vi "Fast_FID_Valve_Control.vi"(7 "Requested Position":T1=1 items=["", "Zero Air", "Calib 1", "Calib 2", "Measure"]) -> (0 "Error Message":string, 3 "Achieved Posn.":T1=1 items=["", "Zero Air", "Calib 1", "Calib 2", "Measure"])   [LabVIEW 2013]
uses:
  Sub VIs/ADAM Controls/Valco_valve_ph.ctl
  Anemometry/Anemometry Sub Vis/Controls/Post_Process.ctl
  Anemometry/Anemometry Sub Vis/Globals/Preference_global.vi
  Anemometry/Anemometry Sub Vis/Globals/Meas_global.vi
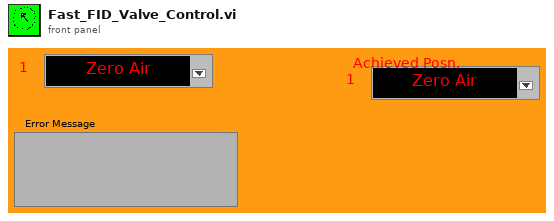
[diagram p1: front panel]
types:
  T1 = typedef "Valco_valve_ph.ctl" = u16
  T2 = typedef "Post_Process.ctl" = enum16{"Take New Data", "Post Process Raw Data File"}
  T3 = typedef "Server_Comms.ctl" = enum16{"Server Link Healthy", "Do Not Link To Server"}
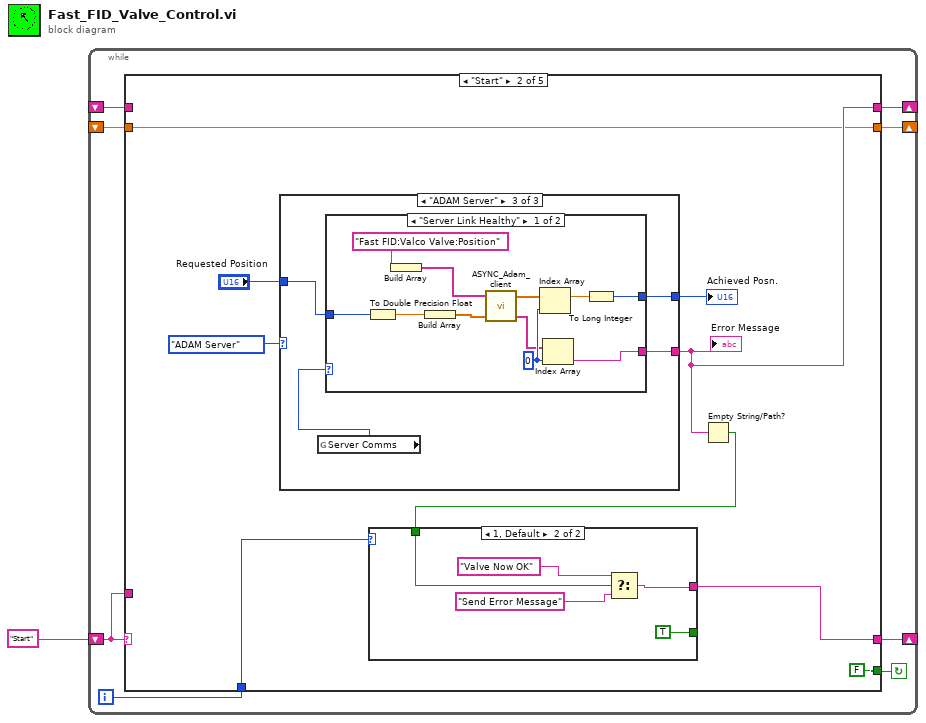
[diagram p0: block diagram]
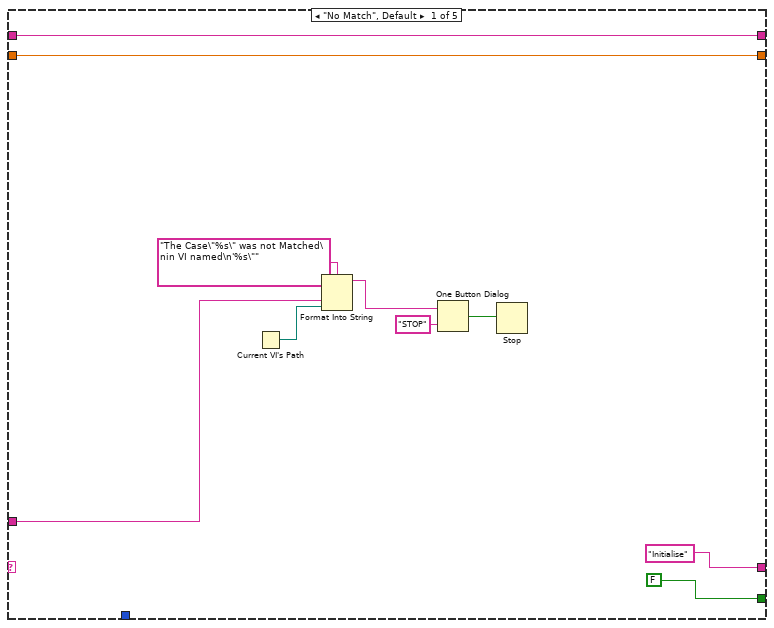
[diagram p2: hidden frame]
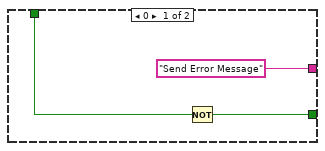
[diagram p3: hidden frame]
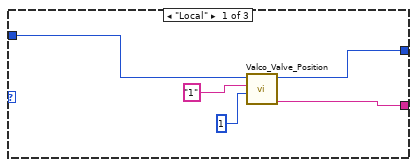
[diagram p4: hidden frame]
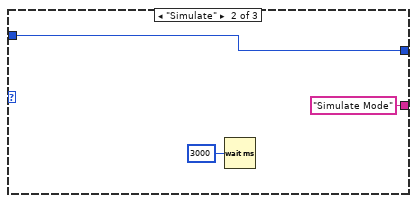
[diagram p5: hidden frame]
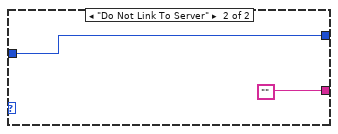
[diagram p6: hidden frame]
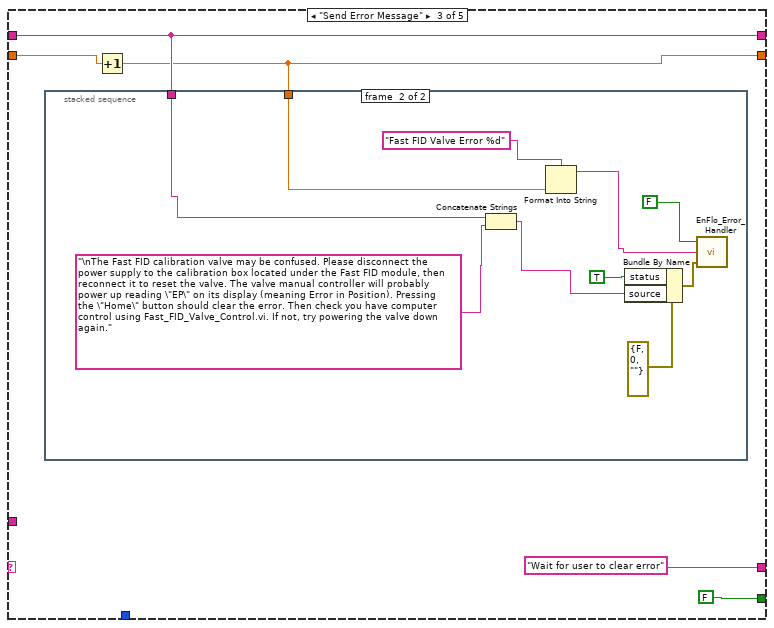
[diagram p7: hidden frame]
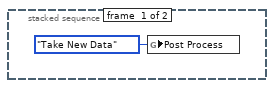
[diagram p8: hidden frame]
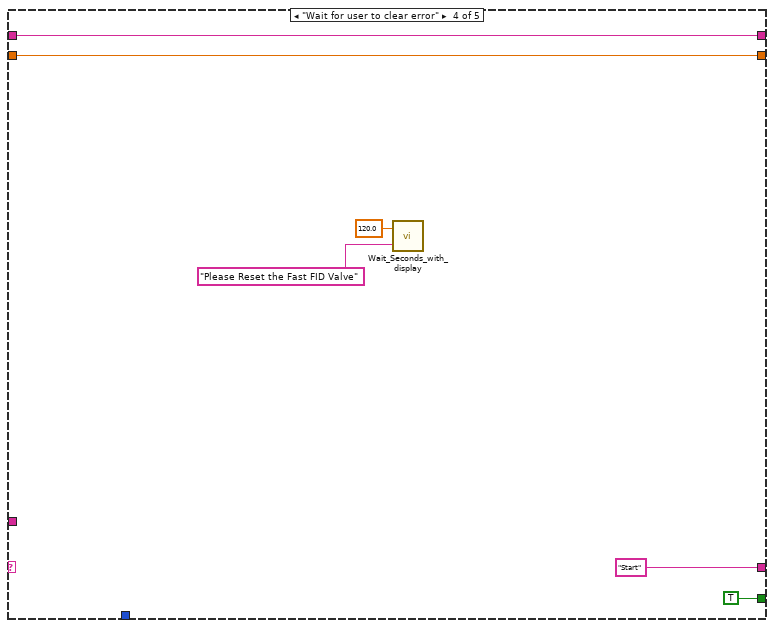
[diagram p9: hidden frame]
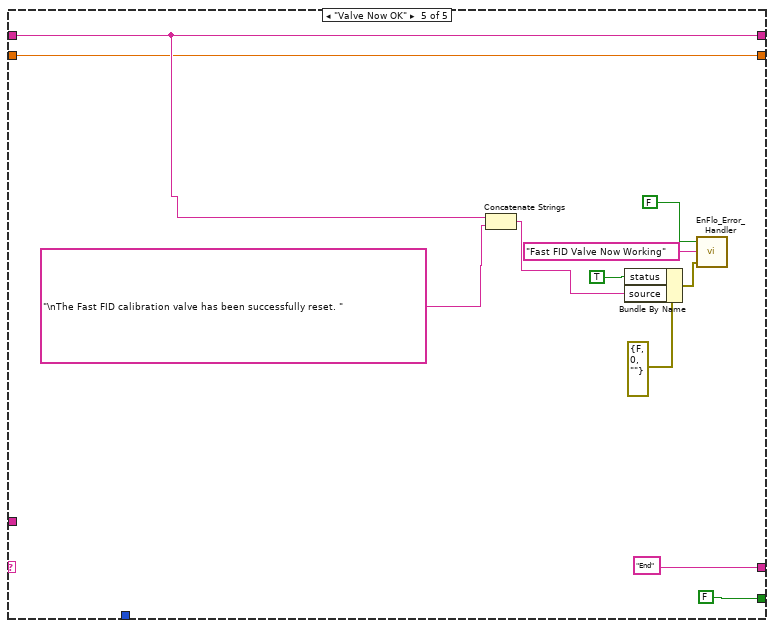
[diagram p10: hidden frame]
diagram:
  n1 = while {
    shift-left: "Start" -> [w7]
    shift-right: [w8] -> _
    shift-right: [w6] -> _
    shift-left: _ -> [w5]
    shift-right: [w2] -> _
    shift-left: _ -> [w3]
    i -> [w4]
    stop <- w9 continue-if-true
    n2 = case shown="\"Start\"" w7 {
      tunnel: [FALSE FALSE FALSE TRUE FALSE] -> w9
      tunnel: ["Initialise" w23 "Wait for user to clear error" "Start" "End"] -> w8
      tunnel: w7 -> [w14 _ _ _ _]
      tunnel: [w11 w26 w64 w80 w85] -> w6
      tunnel: w5 -> [w11 _ w64 w80 w85]
      tunnel: w4 -> [_ w25 _ _ _]
      tunnel: w3 -> [w10 w22 w63 w78 w84]
      tunnel: [w10 w22 w62 w78 w84] -> w2
      frame "No Match", Default {
        n3 = Current VI's Path() -> (path=w13:path)
        n4 = Format Into String(format string="The Case\"%s\" was not Matched\nin VI named\n'%s\"" ("Format String"), w14, w13) -> (resulting string=w17:string)  [unwired: 2 in, 1 out]
        n5 = One Button Dialog(message=w17, button name ("OK")="STOP") -> (true=w15:bool)
        n6 = Stop(stop? (T)=w15) -> ()
      }
      frame "Start" {
        n7 = case shown="\"ADAM Server\"" enum16{"Local", "ADAM Server", "Simulate"}."ADAM Server" ("Case Constant\n(See Context Help)") {
          tunnel: "Requested Position" -> [w40 w44 w48]
          tunnel: [w39 w44 w47] -> w28
          tunnel: [w38 "Simulate Mode" w46] -> w26
          frame "Local" {
            n8 = call "Valco_Valve_Position.vi"("Valve Number"=1, "Port Name"="1", "Requested Posn."=w40) -> ("Error Message"=w38:string, "Achieved Posn."=w39:T1)  [unwired: 1 in, 2 out]
          }
          frame "Simulate" {
            n9 = Wait (ms)(milliseconds to wait=u32 3000) -> ()  [unwired: 1 out]
          }
          frame "ADAM Server" {
            n10 = global read "Preference_global.vi" "Server Comms"() -> (w45:T3)
            n11 = case shown="\"Server Link Healthy\"" w45 {
              tunnel: w48 -> [w51 w61]
              tunnel: [w50 w61] -> w47
              tunnel: [w49 ""] -> w46
              frame "Server Link Healthy" {
                w59 = 0 ("Index")
                n12 = To Double Precision Float(number=w51) -> (double precision float=w54:dbl)
                n13 = Build Array("Fast FID:Valco Valve:Position") -> (w55:string[])
                n14 = Build Array(w54) -> (w56:dbl[])
                n15 = call "ASYNC_Adam_client.vi"("Values"=w56, "Channel Names"=w55) -> ("Scan Comments"=w58:string[], "Calibrated Units"=w57:dbl[])  [unwired: 1 in]
                n16 = Index Array(array=w57, index=w59) -> (element=w53:dbl)
                n17 = Index Array(array=w58, index=w59) -> (element=w49:string)
                n18 = To Long Integer(number=w53) -> (32bit integer=w50:i32)
              }
              frame "Do Not Link To Server" {
              }
            }
          }
        }
        "Error Message" <- w26
        "Achieved Posn." <- w28
        n19 = Empty String/Path?(string/path=w26) -> (empty?=w24:bool)
        n20 = case shown="1, Default" w25 {
          tunnel: w24 -> [w31 w36]
          tunnel: [w30 TRUE] -> _
          tunnel: ["Send Error Message" w34] -> w23
          frame 0 {
            n21 = Not(x=w31) -> (.not. x?=w30:bool)
          }
          frame 1, Default {
            n22 = Select(t="Valve Now OK", s=w36, f="Send Error Message") -> (s? t:f=w34:string)
          }
        }
      }
      frame "Send Error Message" {
        n23 = Increment(x=w63) -> (x+1=w62:dbl)
        n24 = stacked-sequence {
          tunnel: w64 -> [_ w71]
          tunnel: w62 -> [_ w69]
          frame #0 {
            n25 = global write "Meas_global.vi" "Post Process"(Post_Process."Take New Data" ("Post Process")) -> ()
          }
          frame #1 {
            n26 = Concatenate Strings(w71, "\nThe Fast FID calibration valve may be confused. Please disconnect the power supply to the calibration box located under the Fast FID module, then reconnect it to reset the valve. The valve manual controller will probably power up reading \"EP\" on its display (meaning Error in Position). Pressing the \"Home\" button should clear the error. Then check you have computer control using Fast_FID_Valve_Control.vi. If not, try powering the valve down again.") -> (w77:string)
            n27 = Format Into String(format string="Fast FID Valve Error %d" ("Error Type"), w69) -> (resulting string=w68:string)  [unwired: 2 in, 1 out]
            n28 = Bundle By Name(cluster=errorcluster {"status"=FALSE, "code"=0, "source"=""} ("error in (no error)"), "status"=TRUE, "source"=w77) -> (w74:errorcluster)
            n29 = call "EnFlo_Error_Handler.vi"("error in (no error)"=w74, "Error Type"=w68, "Dialog Box (T)"=FALSE) -> ()  [unwired: 3 out]
          }
        }
      }
      frame "Wait for user to clear error" {
        n30 = call "Wait_Seconds_with_display.vi"("Message"="Please Reset the Fast FID Valve", "Seconds to wait"=120.0) -> ()  [unwired: 2 out]
      }
      frame "Valve Now OK" {
        n31 = Concatenate Strings(w85, "\nThe Fast FID calibration valve has been successfully reset. ") -> (w92:string)
        n32 = Bundle By Name(cluster=errorcluster {"status"=FALSE, "code"=0, "source"=""} ("error in (no error)"), "status"=TRUE, "source"=w92) -> (w89:errorcluster)
        n33 = call "EnFlo_Error_Handler.vi"("error in (no error)"=w89, "Error Type"="Fast FID Valve Now Working", "Dialog Box (T)"=FALSE) -> ()  [unwired: 3 out]
      }
    }
  }
